vi "niDTS CommLib Path.vi"() -> (3 "CommLib Path":path)   [LabVIEW 2015, in "niDTS CommLib.lvlib"]
uses:
  niDTS CommLib.lvlib
  Framework/Comm/Objects/BASE_class/niDTS Comm.lvclass
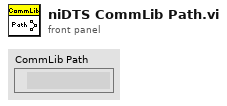
[diagram p1: front panel]
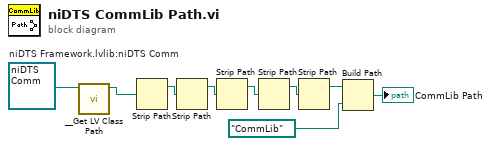
[diagram p0: block diagram]
diagram:
  w9 = refnum<class "niDTS Comm.lvclass"> refnum  # niDTS Framework.lvlib:niDTS Comm
  n1 = call "__Get LV Class Path.vi"("object"=w9) -> ("class path"=w8:path)  [unwired: 9 in, 1 out]
  n2 = Strip Path(path=w8) -> (stripped path=w7:path)  [unwired: 1 out]
  n3 = Strip Path(path=w7) -> (stripped path=w6:path)  [unwired: 1 out]
  n4 = Strip Path(path=w6) -> (stripped path=w4:path)  [unwired: 1 out]
  n5 = Strip Path(path=w4) -> (stripped path=w5:path)  [unwired: 1 out]
  n6 = Strip Path(path=w5) -> (stripped path=w3:path)  [unwired: 1 out]
  n7 = Build Path(base path=w3, name or relative path=path "CommLib") -> (appended path=→"CommLib Path":path)
